vi "Wait until time.vi"(9 "Initial Time":timestamp, 10 "Time to wait for":dbl, 11 "Run?":bool) -> (3 "Done":bool)   [LabVIEW 2013]
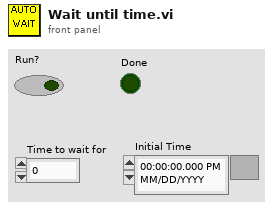
[diagram p1: front panel]
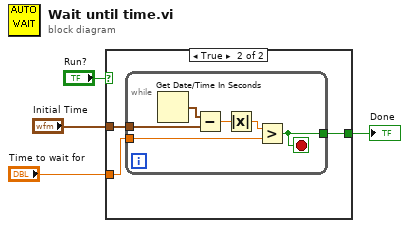
[diagram p0: block diagram]
diagram:
  n1 = case shown="True" "Run?" {
    selector: "Run?" -> [w5 _]
    tunnel: [w5 w7] -> w3
    tunnel: "Time to wait for" -> [_ w8]
    tunnel: "Initial Time" -> [_ w6]
    frame False {
    }
    frame True {
      n2 = while {
        tunnel: w8 -> [w14]
        tunnel: [w13] -> w7
        tunnel: w6 -> [w9]
        stop <- w13 stop-if-true
        n3 = Get Date/Time In Seconds() -> (seconds since 1Jan1904=w10:timestamp)
        n4 = Subtract(x=w10, y=w9) -> (x-y=w11:dbl)
        n5 = Absolute Value(x=w11) -> (abs(x)=w12:dbl)
        n6 = Greater?(x=w12, y=w14) -> (0:w13:bool)
      }
    }
  }
  "Done" <- w3
